vi "gRPC Data Transfer.vi"(6 "Main to gRPC":T2, 11 "Node in":refnum<class "ThermotronDriver.lvclass">) -> (1 "Update":bool, 3 "Node out":refnum<class "ThermotronDriver.lvclass">, 4 "gRPC to Main":T1)   [LabVIEW 2023, in "ThermotronDriver.lvlib" / "ThermotronDriver.lvclass"]
uses:
  ThermotronDriver.lvclass
  Out Of Band/Type Defs/Main to gRPC.ctl
  Out Of Band/Type Defs/gRPC to Main.ctl
  Out Of Band/gRPC Loop/Class to gRPC_to_Main.vi
  ThermotronDriver.lvclass/ThermotronDriver.ctl
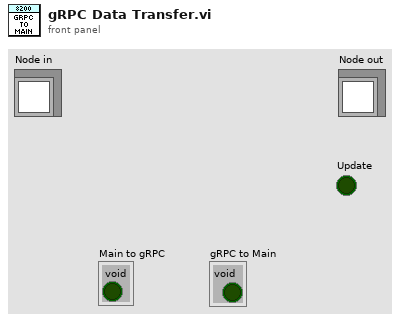
[diagram p1: front panel]
types:
  T1 = typedef "ThermotronDriver.lvlib/ThermotronDriver.lvclass/gRPC to Main.ctl" = cluster{"void":bool}
  T2 = typedef "ThermotronDriver.lvlib/ThermotronDriver.lvclass/Main to gRPC.ctl" = cluster{"void":bool}
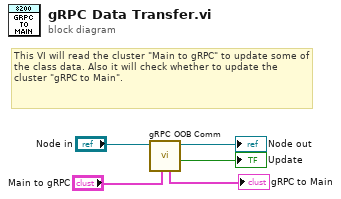
[diagram p0: block diagram]
diagram:
  # "This VI will read the cluster \"Main to gRPC\" to update some of the class data. Also it will check whether to update the cluster \"gRPC to Main\"."
  n1 = call "gRPC OOB Comm.vi"("Main to gRPC"="Main to gRPC", "Node in"="Node in") -> ("Update gRPC"=→"Update":bool, "Node out"=→"Node out":refnum<class "ThermotronDriver.lvclass">, "gRPC to Main"=→"gRPC to Main":T1)  [unwired: 7 in]
